vi "WasRun_Create.vi"(8 "error in (no error)":errorcluster, 10 "Name":string) -> (0 "error out":errorcluster, 3 "WasRun out":refnum<class "WasRun.lvclass">)   [LabVIEW 2013, in "WasRun.lvclass"]
uses:
  WasRun.lvclass
  WasRun.lvclass/WasRun.ctl
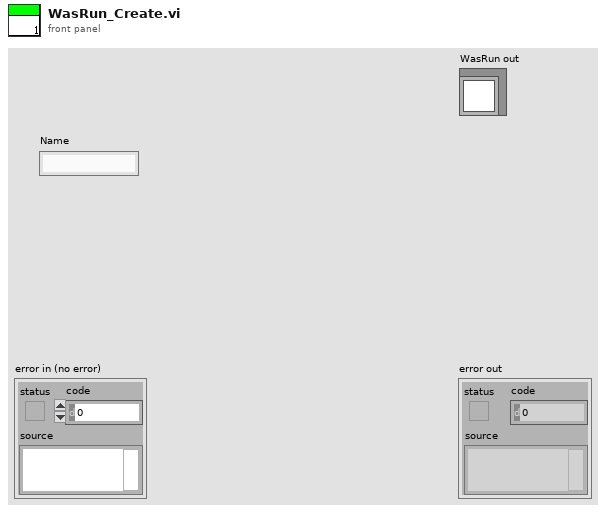
[diagram p1: front panel]
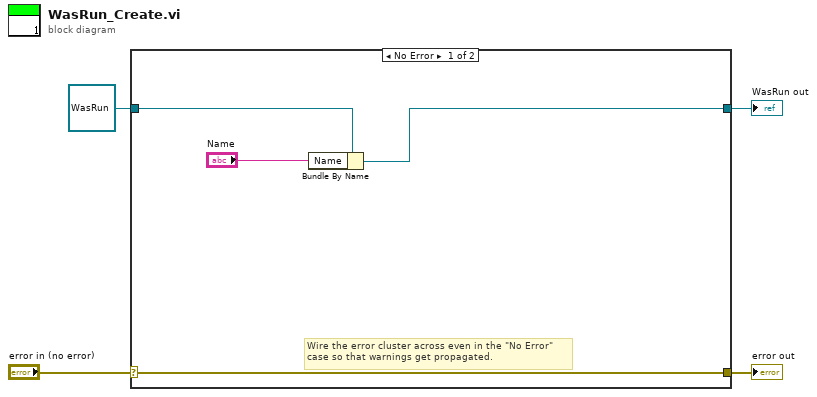
[diagram p0: block diagram]
diagram:
  n1 = case shown="No Error" "error in (no error)" {
    selector: "error in (no error)" -> [w8 w10]
    tunnel: [w8 w10] -> w3
    tunnel: [w5 w9] -> w1
    tunnel: refnum<class "WasRun.lvclass"> refnum ("WasRun in") -> [w6 w9]
    frame No Error {
      # "Wire the error cluster across even in the \"No Error\"\ncase so that warnings get propagated."
      n2 = Bundle By Name(cluster=w6, "Name"="Name") -> (w5:refnum<class "WasRun.lvclass">)
    }
    frame Error {
    }
  }
  "error out" <- w3
  "WasRun out" <- w1
